vi "Anangram.vi"(6 "EXIT":bool, 7 "ANAGRAM?":bool, 8 "error in":errorcluster, 10 "STRING 2":string, 11 "STRING 1":string) -> (0 "error out":errorcluster)   [LabVIEW 2020]
doc: "An anagram is a word or phrase formed by rearranging the letters of a different word or phrase, typically using all the original letters exactly once.\n\nThis VI is built using Simple Event Driven State Machine Design Pattern."
uses:
  Enum.ctl
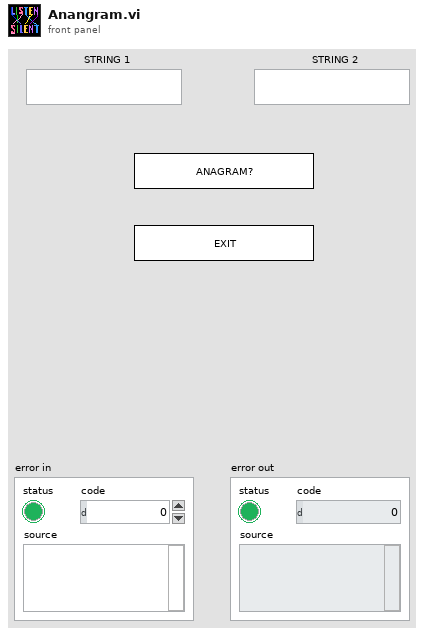
[diagram p1: front panel]
types:
  T1 = typedef "Enum.ctl" = enum16{"Initialize", "Main", "Error Handling", "Exit"}
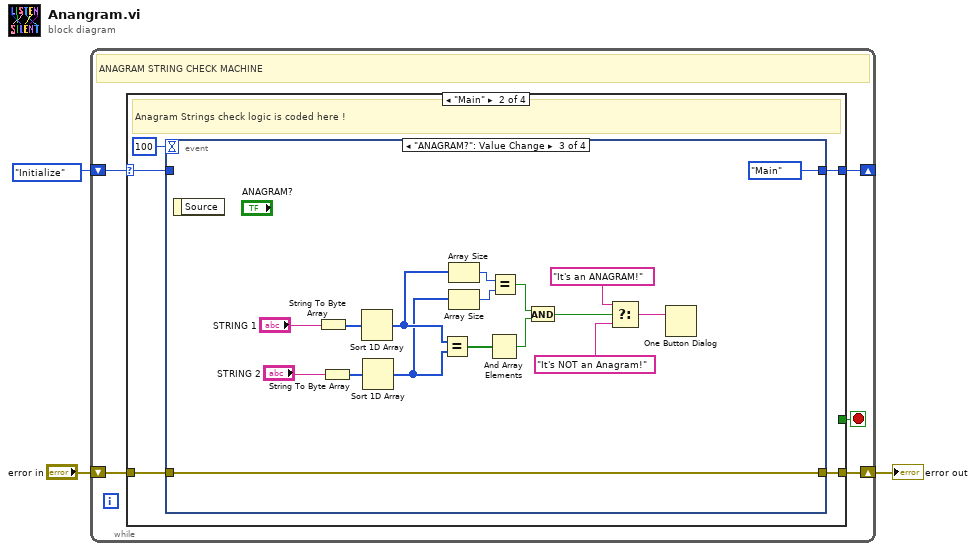
[diagram p0: block diagram]
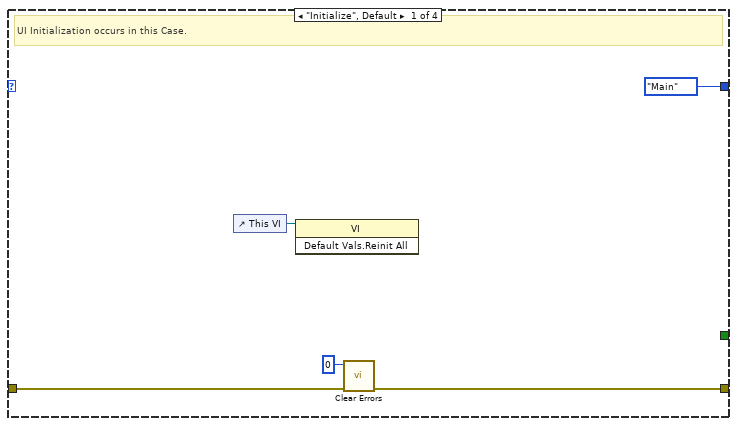
[diagram p2: hidden frame]
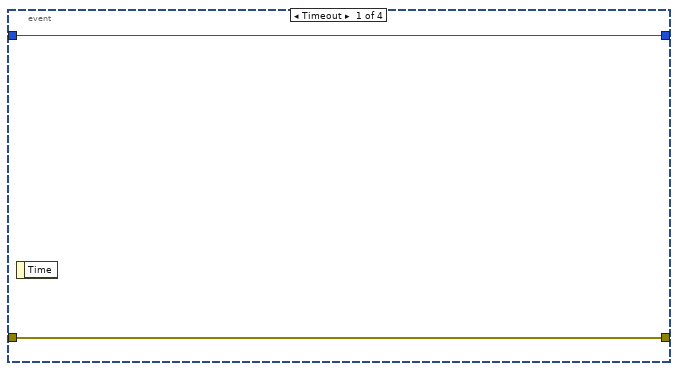
[diagram p3: hidden frame]
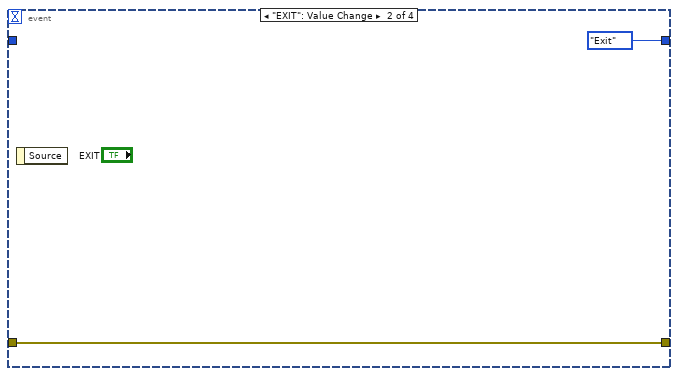
[diagram p4: hidden frame]
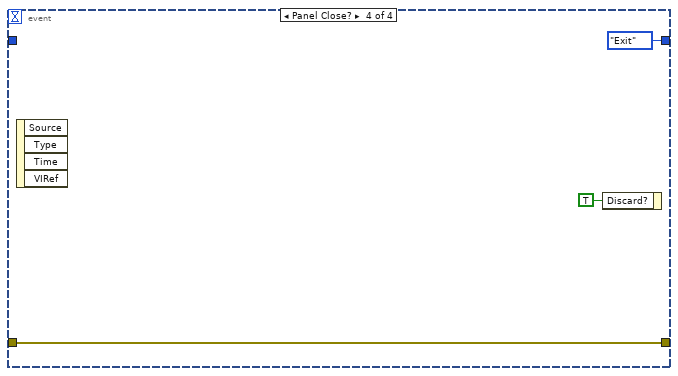
[diagram p5: hidden frame]
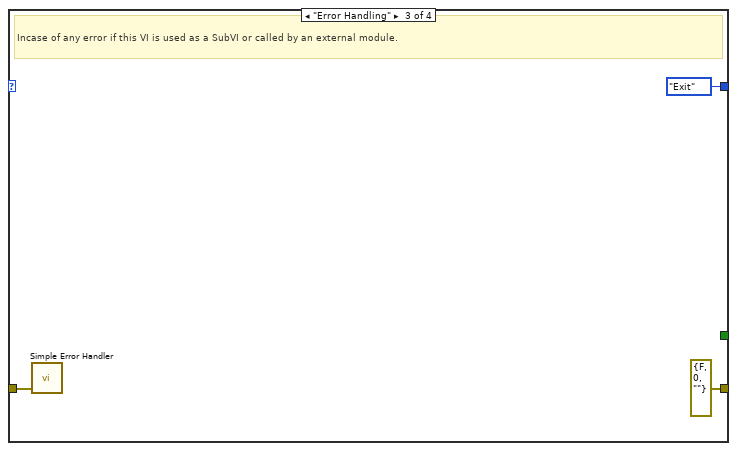
[diagram p6: hidden frame]
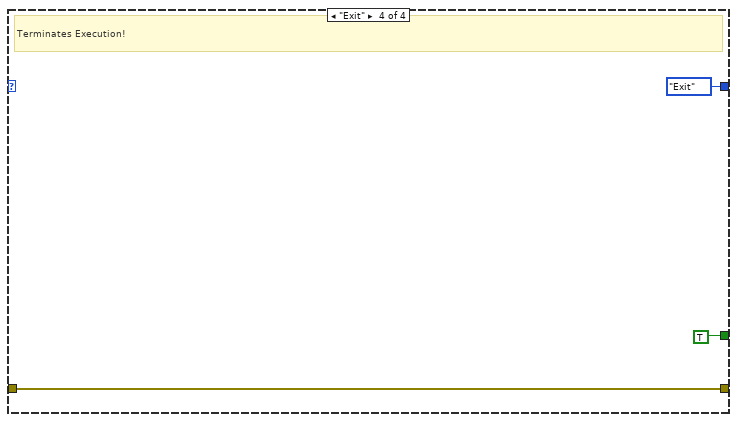
[diagram p7: hidden frame]
diagram:
  n1 = while {
    shift-right: [w7] -> _
    shift-left: Enum."Initialize" -> [w8]
    shift-right: [w5] -> w1
    shift-left: "error in" -> [w6]
    stop <- w4 stop-if-true
    # "ANAGRAM STRING CHECK MACHINE"
    n2 = case shown="\"Main\"" w8 {
      selector: w8 -> [_ w14 _ _]
      tunnel: [Enum."Main" w15 Enum."Exit" Enum."Exit"] -> w7
      tunnel: w6 -> [w11 w17 w45 w46]
      tunnel: [w9 w16 errorcluster {"status"=FALSE, "code"=0, "source"=""} ("error in") w46] -> w5
      tunnel: [_ _ _ TRUE] -> w4
      frame "Initialize", Default {
        # "UI Initialization occurs in this Case."
        n3 = control-ref of="This VI"() -> (w12:refnum<vi>)
        n4 = invoke class="VI" method="Default Vals.Reinit All"(reference=w12) -> ()  [unwired: 2 in, 3 out]
        n5 = call <vilib>:"Clear Errors.vi"("error in (no error)"=w11, "specific error code to clear (0: all)"=0) -> ("error out"=w9:errorcluster)  [unwired: 4 in, 1 out]
      }
      frame "Main" {
        # "Anagram Strings check logic is coded here !"
        n6 = event shown="[2] \"ANAGRAM?\": Value Change" {
          selector: _ -> [_ _ _ _]
          dyn-events: _ -> [_ _ _ _]
          timeout: 100 -> [_ _ _ _]
          tunnel: w17 -> [w20 w22 w39 w42]
          tunnel: [w20 w22 w39 w42] -> w16
          tunnel: [w19 Enum."Exit" Enum."Main" Enum."Exit"] -> w15
          tunnel: w14 -> [w19 _ _ _]
          event Timeout {
            n7 = event-data() -> ()  [unwired: 1 in, 1 out]
          }
          event "EXIT": Value Change {
            n8 = event-data() -> ()  [unwired: 1 in, 1 out]
          }
          event "ANAGRAM?": Value Change {
            n9 = event-data() -> ()  [unwired: 1 in, 1 out]
            n10 = String To Byte Array(string="STRING 1") -> (unsigned byte array=w35:u8[])
            n11 = String To Byte Array(string="STRING 2") -> (unsigned byte array=w34:u8[])
            n12 = Sort 1D Array(array=w35) -> (sorted array=w32:u8[])
            n13 = Sort 1D Array(array=w34) -> (sorted array=w31:u8[])
            n14 = Equal?(x=w32, y=w31) -> (x = y?=w33:bool[])
            n15 = Array Size(array=w32) -> (size(s)=w30:i32)
            n16 = Array Size(array=w31) -> (size(s)=w29:i32)
            n17 = And Array Elements(Boolean array=w33) -> (logical AND=w27:bool)
            n18 = Equal?(x=w30, y=w29) -> (x = y?=w28:bool)
            n19 = And(x=w28, y=w27) -> (x .and. y?=w26:bool)
            n20 = Select(t="It's an ANAGRAM!", s=w26, f="It's NOT an Anagram!") -> (s? t:f=w23:string)
            n21 = One Button Dialog(message=w23) -> ()  [unwired: 1 in, 1 out]
          }
          event Panel Close? {
            n22 = event-data() -> ()  [unwired: 1 in, 4 out]
            n23 = event-data("Discard?"=TRUE) -> ()  [unwired: 1 in, 1 out]
          }
        }
      }
      frame "Error Handling" {
        # "Incase of any error if this VI is used as a SubVI or called by an external module."
        n24 = call <vilib>:"Simple Error Handler.vi"("error in (no error)"=w45) -> ()  [unwired: 4 in, 5 out]
      }
      frame "Exit" {
        # "Terminates Execution!"
      }
    }
  }
  "error out" <- w1
